vi "thcd401_format_data.vi"(8 "index":i32, 9 "mode_array":i32[](array[numeric]), 10 "value_array":dbl[](array[numeric]), 11 "time":timestamp) -> (0 "mode":i32, 1 "value":dbl, 3 "waveform_array":waveform(dbl)[](array[waveform])=[{"t0"=timestamp(0 s since 1904-01-01), "dt"=1.0, "Y"=[]}, {"t0"=timestamp(3732035173.078092 s since 1904-01-01), "dt"=1.0, "Y"=[302.8589782714844], "attributes"=variant("NI_ChannelName"=variant(string "T1"))}], 4 "mode_str":string)   [LabVIEW 2019]
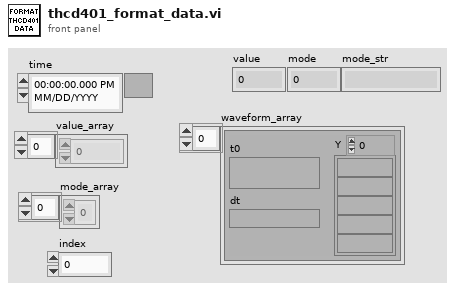
[diagram p1: front panel]
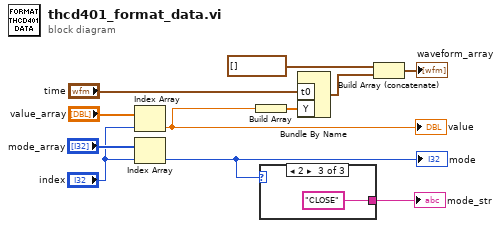
[diagram p0: block diagram]
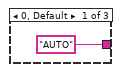
[diagram p2: hidden frame]
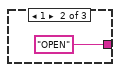
[diagram p3: hidden frame]
diagram:
  n1 = Index Array(array="value_array", index="index") -> (element=w5:dbl)
  "value" <- w5
  n2 = Index Array(array="mode_array", index="index") -> (element=w2:i32)
  "mode" <- w2
  n3 = Build Array(w5) -> (w10:dbl[])
  n4 = case shown="2" w2 {
    tunnel: ["AUTO" "OPEN" "CLOSE"] -> w1
    frame 0, Default {
    }
    frame 1 {
    }
    frame 2 {
    }
  }
  "mode_str" <- w1
  n5 = Bundle By Name("t0"="time", "Y"=w10) -> (w9:waveform(dbl))  [unwired: 1 in]
  n6 = Build Array (concatenate)(waveform(dbl)[] [], w9) -> (→"waveform_array":waveform(dbl)[])
